vi "Shutter_OpenIfClosed.vi"(0 "KCube Shutter Device Reference 2":refnum<vi>, 1 "Shutter Ctrls 2":refnum<vi>, 2 "Shutter on?":bool) -> ()   [LabVIEW 2019]
uses:
  D:/Users/manip-thz/Documents/Controle_Manip_2020/Thorlabs.MotionControl.KCube.SolenoidCLI.dll
  Thorlabs.MotionControl.KCube.SolenoidCLI.dll
panel:
  in  "KCube Shutter Device Reference":refnum<k24>
  in  "Shutter Ctrls":u16(ring)
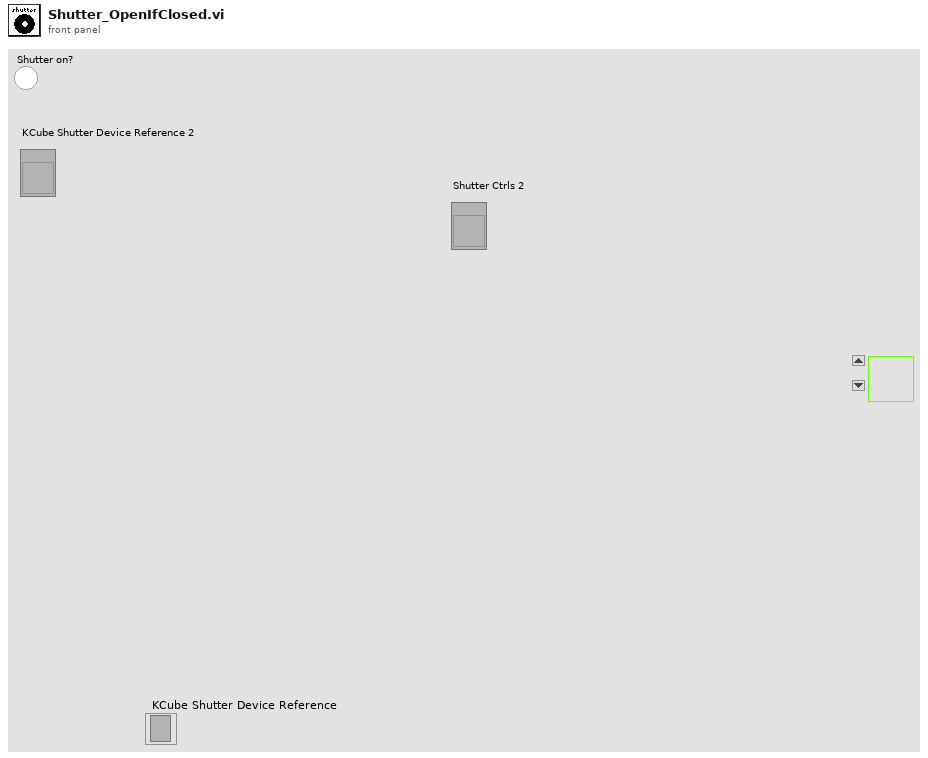
[diagram p1: front panel]
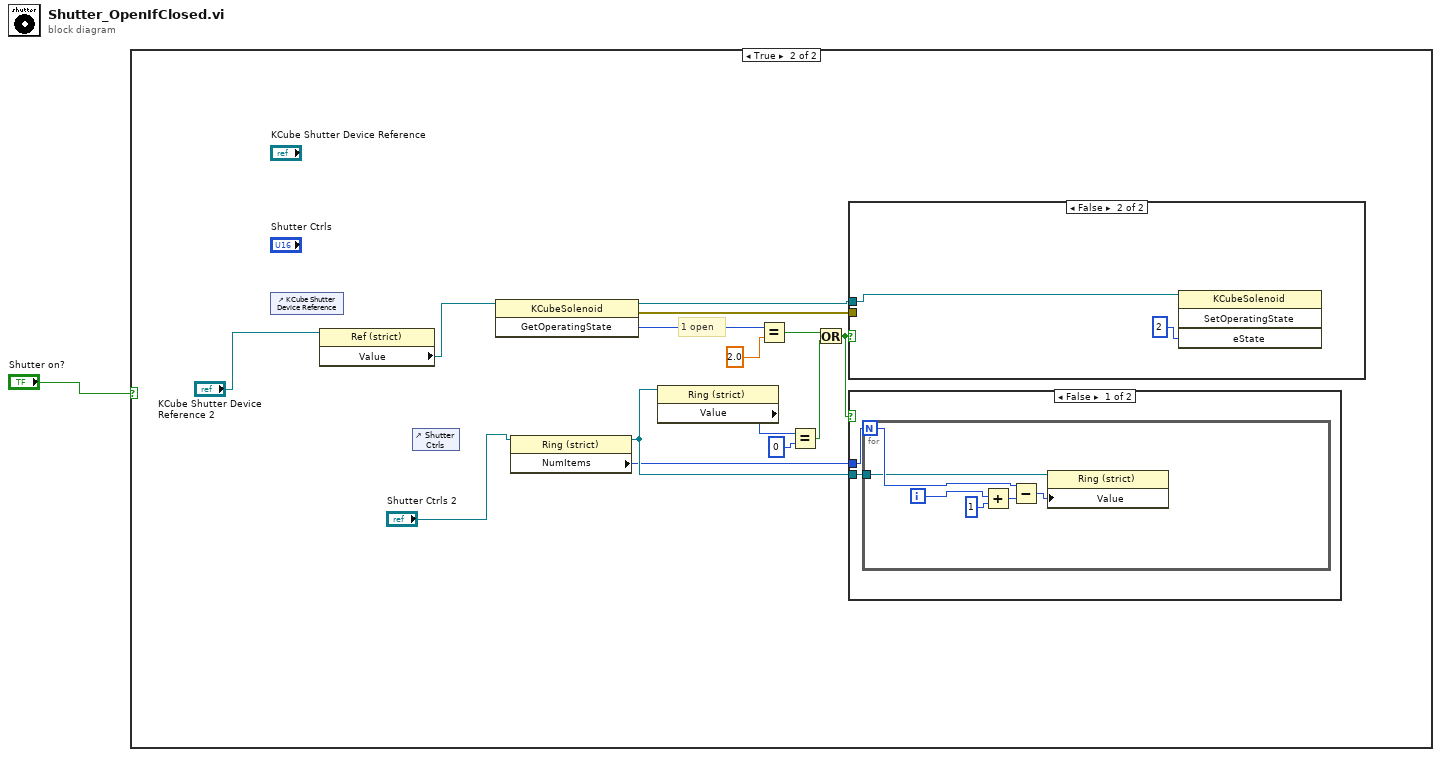
[diagram p0: block diagram]
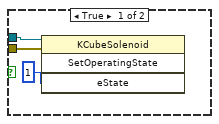
[diagram p3: hidden frame]
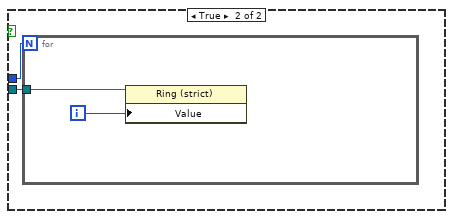
[diagram p4: hidden frame]
diagram:
  n1 = case shown="True" "Shutter on?" {
    frame False {
    }
    frame True {
      # "1 open"
      n2 = control-ref of="KCube Shutter Device Reference"() -> ()  [unwired: 1 out]
      n3 = property class="Ref (strict)"(reference="KCube Shutter Device Reference 2") -> ("Value"=w4:refnum<k24>)  [unwired: 1 in, 2 out]
      n4 = control-ref of="Shutter Ctrls"() -> ()  [unwired: 1 out]
      n5 = invoke class="KCubeSolenoid" method="GetOperatingState"(reference=w4) -> (reference out=w14:refnum<k24>, error out=w15:errorcluster, "GetOperatingState"=w13:i32)  [unwired: 2 in]
      n6 = property on="Property Node" class="Ring (strict)"(reference="Shutter Ctrls 2") -> (reference out=w6:refnum<vi>, "NumItems"=w5:u32)  [unwired: 1 in, 1 out]
      n7 = property on="Property Node" class="Ring (strict)"(reference=w6) -> ("Value"=w7:u16)  [unwired: 1 in, 2 out]
      n8 = Equal?(x=w13, y=2.0) -> (x = y?=w9:bool)
      n9 = Equal?(x=w7, y=u16 0) -> (x = y?=w10:bool)
      n10 = Or(x=w9, y=w10) -> (x .or. y?=w11:bool)
      n11 = case shown="False" w11 {
        tunnel: w14 -> [w17 w19]
        tunnel: w15 -> [w16 _]
        frame True {
          n12 = invoke class="KCubeSolenoid" method="SetOperatingState"(reference=w17, error in=w16, "eState"=1) -> ()  [unwired: 1 in, 4 out]
        }
        frame False {
          n13 = invoke class="KCubeSolenoid" method="SetOperatingState"(reference=w19, "eState"=2) -> ()  [unwired: 2 in, 4 out]
        }
      }
      n14 = case shown="False" w11 {
        tunnel: w5 -> [w21 w30]
        tunnel: w6 -> [w22 w29]
        frame False {
          n15 = for {
            N: w21 -> [w28]
            tunnel: w22 -> [w26]
            i -> [w27]
            n16 = Add(x=w27, y=1) -> (x+y=w24:i32)
            n17 = Subtract(x=w28, y=w24) -> (x-y=w25:i32)
            n18 = property on="Property Node" class="Ring (strict)"(reference=w26, "Value"=w25) -> ()  [unwired: 1 in, 2 out]
          }
        }
        frame True {
          n19 = for {
            N: w30 -> [_]
            tunnel: w29 -> [w31]
            i -> [w32]
            n20 = property on="Property Node" class="Ring (strict)"(reference=w31, "Value"=w32) -> ()  [unwired: 1 in, 2 out]
          }
        }
      }
    }
  }
